vi "Generate Handle Error Event.vi"(6 "UsrEvtRef":refnum<user-event>, 8 "error in":errorcluster) -> ()   [LabVIEW 2025]
uses:
  <vilib>/event_ctls.llb/usereventprio.ctl
  cmd-data event messenger/source/Event Data.ctl
  cmd-data event messenger/source/Cmd-Data Event Messenger.lvlib
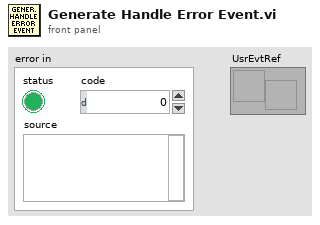
[diagram p1: front panel]
types:
  T1 = typedef "Cmd-Data Event Messenger.lvlib/Event Data.ctl" = cluster{"msg":cluster{"cmd":string, "data":variant}, "valid?":bool, "last?":bool, "aborted?":bool, "priority?":bool}
  T2 = typedef "usereventprio.ctl" = enum32{"high priority", "normal priority"}
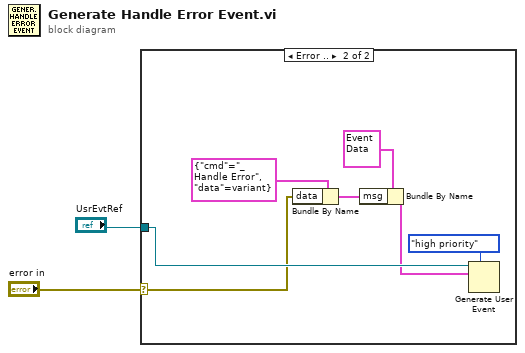
[diagram p0: block diagram]
diagram:
  n1 = case shown="Error .." "error in" {
    selector: "error in" -> [_ w7]
    tunnel: "UsrEvtRef" -> [_ w8]
    frame No Error {
    }
    frame Error {
      n2 = Bundle By Name(cluster=cluster{"cmd":string, "data":variant} {"cmd"="_Handle Error", "data"=variant} ("element"), "data"=w7) -> (w6:cluster{"cmd":string, "data":variant})
      n3 = Bundle By Name(cluster=T1 {"msg"={"cmd"="", "data"=variant}, "valid?"=FALSE, "last?"=FALSE, "aborted?"=FALSE, "priority?"=FALSE} ("event data"), "msg"=w6) -> (w3:T1)
      n4 = Generate User Event(priority (normal)=usereventprio."high priority", user event=w8, event data cluster=w3) -> ()  [unwired: 1 in, 2 out]
    }
  }
